vi "Begin.vi"(8 "error in":errorcluster) -> (0 "error out":errorcluster)   [LabVIEW 2015]
doc: "Called before other user functions, this VI is expected to open initial I/O refnums, load in file data, and do all program initialization. Notice that the <B>error out</B> terminal is simply used for data flow. Wiring it to other structures or subVIs ensures that this VI runs first."
uses:
  <vilib>/Rock Robotics/SystemInterfaces/DIO/FPGA_DIOPWMChannel.ctl
  <vilib>/Rock Robotics/WPI/DriverStation/WPI_DriverStationRobotMode2.ctl
  <vilib>/Rock Robotics/WPI/Joystick/WPI_JoystickDeviceEnum.ctl
  <vilib>/Rock Robotics/SystemInterfaces/AI/FPGA_AIChannel.ctl
  <vilib>/Rock Robotics/WPI/SafetyOutput/WPI_SafetyOutputConfigMenu.ctl
  <vilib>/Rock Robotics/SystemInterfaces/DIO/FPGA_DIOChannel.ctl
  <vilib>/Rock Robotics/WPI/Solenoid/WPI_SolenoidChannel.ctl
  <vilib>/Rock Robotics/SystemInterfaces/spilib/spi_bus.ctl
  <vilib>/Rock Robotics/WPI/RobotDrive/WPI_RobotDriveOpen2MotorWithSPARK.vi
  Robot Global Data.vi
  <vilib>/Rock Robotics/Network Tables/NT Write String Array.vi
  <vilib>/Rock Robotics/WPI/MotorControl/WPI_MotorControlOpen SPARK.vi
  <vilib>/Rock Robotics/WPI/Counter/WPI_CounterDigitalInputToDigitalSource.vi
  <vilib>/Rock Robotics/WPI/Solenoid/WPI_SolenoidOpenDouble.vi
  NavX/navX Library v2.lvlib
  ArmController/ArmController.lvlib
  <vilib>/Rock Robotics/WPI/Solenoid/WPI_SolenoidSetEnum.vi
  <vilib>/Rock Robotics/WPI/Solenoid/WPI_SolenoidValue.ctl
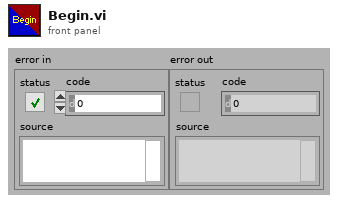
[diagram p1: front panel]
types:
  T1 = typedef "WPI_SafetyOutputConfigMenu.ctl" = enum16{"Enable", "Disable"}
  T2 = typedef "WPI_SolenoidChannel.ctl" = enum8{"Solenoid 0", "Solenoid 1", "Solenoid 2", "Solenoid 3", "Solenoid 4", "Solenoid 5", "Solenoid 6", "Solenoid 7", "Invalid"}
  T3 = typedef "FPGA_DIOChannel.ctl" = enum8{"DIO 0", "DIO 1", "DIO 2", "DIO 3", "DIO 4", "DIO 5", "DIO 6", "DIO 7", "DIO 8", "DIO 9", "DIO MXP 0", "DIO MXP 1", "DIO MXP 2", "DIO MXP 3", "DIO MXP 4", "DIO MXP 5", "DIO MXP 6", "DIO MXP 7", "DIO MXP 8", "DIO MXP 9", "DIO MXP 10", "DIO MXP 11", "DIO MXP 12", "DIO MXP 13", "DIO MXP 14", "DIO MXP 15", "Invalid"}
  T4 = typedef "FPGA_AIChannel.ctl" = enum8{"AI 0", "AI 1", "AI 2", "AI 3", "AI MXP 0", "AI MXP 1", "AI MXP 2", "AI MXP 3", "Invalid"}
  T5 = cluster{"proportional gain (Kc)":dbl, "integral time (Ti, min)":dbl, "derivative time (Td, min)":dbl}
  T6 = typedef "FPGA_DIOPWMChannel.ctl" = enum8{"PWM 0", "PWM 1", "PWM 2", "PWM 3", "PWM 4", "PWM 5", "PWM 6", "PWM 7", "PWM 8", "PWM 9", "PWM MXP 0", "PWM MXP 1", "PWM MXP 2", "PWM MXP 3", "PWM MXP 4", "PWM MXP 5", "PWM MXP 6", "PWM MXP 7", "PWM MXP 8", "PWM MXP 9", "Invalid"}
  T7 = typedef "WPI_JoystickDeviceEnum.ctl" = enum16{"USB 0", "USB 1", "USB 2", "USB 3", "USB 4", "USB 5"}
  T8 = typedef "WPI_DriverStationRobotMode2.ctl" = enum16{"Autonomous Disabled", "Autonomous Enabled", "Teleop Disabled", "Teleop Enabled", "Disconnected", "Finish", "Test Disabled", "Test Enabled", "Emergency Stopped"}
  T9 = typedef "WPI_SolenoidValue.ctl" = enum16{"Off", "On", "Forward", "Reverse"}
  T10 = typedef "WPI_RobotDriveDevRef.ctl" = cluster{"DevStatus":errorcluster, "Motors[]":T11[], "Square Inputs":bool, "Max Output":dbl}
  T11 = typedef "WPI_MotorControlDeviceRef.ctl" = cluster{"DeviceStatus":errorcluster, "Type":T12, "PWM":cluster{"PWM Channel":T6, "DeadBand":T13}, "CAN":cluster{"Device Number":u8, "Control Mode":T14, "Semaphore":T15, "Max Vout":dbl, "TalonSRX Control Mode":T16}, "Invert":bool}
  T12 = typedef "WPI_MotorControlType.ctl" = enum16{"PWM", "CAN", "CANTalonSRX"}
  T13 = typedef "WPI_PWMDeadband.ctl" = cluster{"Name":string, "maxPositivePwm":i32, "minPositivePwm":i32, "centerPwm":i32, "maxNegativePwm":i32, "minNegativePwm":i32, "angularRange":u16}
  T14 = typedef "WPI_CANJaguar_ControlMode.ctl" = enum8{"Percent VBus", "Current", "Speed", "Position", "Voltage"}
  T15 = typedef "Semaphore RefNum" = refnum<k1>
  T16 = typedef "WPI_CANTalonSRX_APIControlMode.ctl" = enum8{"Percent VBus", "Speed", "Position", "Slave", "Unchanged / Invalid", "Voltage Compensation", "Current", "Motion Profile"}
  T17 = typedef "WPI_SolenoidDevRef.ctl" = cluster{"DevStatus":errorcluster, "Pneumatics Control Module":u8, "Forward Solenoid Channel":T2, "Reverse Solenoid Channel":T2}
  T18 = typedef "WPI_ServoDeviceRef.ctl" = cluster{"DeviceStatus":errorcluster, "PWM Channel":T6, "DeadBand":T13}
  T19 = typedef "WPI_JoystickDevRef.ctl" = cluster{"Device":T7}
  T20 = typedef "spi_bus.ctl" = enum16{"SPI On-Board, CS0", "SPI On-Board, CS1", "SPI On-Board, CS2", "SPI On-Board, CS3", "SPI MXP", "Invalid"}
  T21 = typedef "navX Library v2.lvlib/Z900_navX_DeviceTypeDef.ctl" = cluster{"Interface":cluster{"Protocol":T22, "Update Rate (4Hz-60Hz)":u8, "navX Open TypeDef":variant}, "Notify Packet":refnum<notifier>, "Loop VI Refnum":refnum<vi>, "Ready to Close Occurrence Refnum":refnum<k4>}
  T22 = typedef "navX Library v2.lvlib/Z900_navX_ProtocolTypeDef.ctl" = enum16{"SERIAL", "I2C", "SPI"}
  T23 = typedef "WPI_DigitalInputDevRef.ctl" = cluster{"DevStatus":errorcluster, "DIO Channel":T3}
  T24 = typedef "FPGA_CounterEncoderSourceConvertionLVSourceType.ctl" = cluster{"DevStatus":errorcluster, "AnalogTriggerMode?":bool, "DigitalMode":cluster{"DIO Channel":T25}, "AnalogTriggerMode":cluster{"AnalogTriggerIndex":T26, "OutputType":T27}}
  T25 = typedef "FPGA_DIODigitalSourceChannel.ctl" = enum8{"DIO 0", "DIO 1", "DIO 2", "DIO 3", "DIO 4", "DIO 5", "DIO 6", "DIO 7", "DIO 8", "DIO 9", "DIO MXP 0", "DIO MXP 1", "DIO MXP 2", "DIO MXP 3", "DIO MXP 4", "DIO MXP 5", "DIO MXP 6", "DIO MXP 7", "DIO MXP 8", "DIO MXP 9", "DIO MXP 10", "DIO MXP 11", "DIO MXP 12", "DIO MXP 13", "DIO MXP 14", "DIO MXP 15", "Disabled"}
  T26 = typedef "FPGA_AnalogTriggerIndex.ctl" = enum8{"Trig 0", "Trig 1", "Trig 2", "Trig 3", "Trig 4", "Trig 5", "Trig 6", "Trig 7", "Invalid"}
  T27 = typedef "FPGA_AnalogTriggerOutType.ctl" = enum16{"InWindow", "TriggerState", "Rising", "Falling"}
  T28 = typedef "WPI_EncoderDevRef.ctl" = cluster{"DevStatus":errorcluster, "EncoderIndex":T29, "CounterIndex":T30, "DistancePerCount":dbl, "Decoding Type":T31}
  T29 = typedef "FPGA_EncoderIdx.ctl" = enum8{"Enc 0", "Enc 1", "Enc 2", "Enc 3", "Enc 4", "Enc 5", "Enc 6", "Enc 7", "Invalid"}
  T30 = typedef "FPGA_CounterCtrSystemIndex.ctl" = enum8{"Ctr 0", "Ctr 1", "Ctr 2", "Ctr 3", "Ctr 4", "Ctr 5", "Ctr 6", "Ctr 7", "Invalid"}
  T31 = typedef "WPI_EncoderType.ctl" = enum16{"1x", "2x", "4x"}
  T32 = typedef "WPI_PotentiometerDevRef.ctl" = cluster{"DevStatus":errorcluster, "Analog Channel":T4, "Invert Output":bool}
  T33 = typedef "ArmController.lvlib/ArmRef.ctl" = cluster{"Pot":T32, "ArmMotor":T11, "Queue":refnum<queue>, "Setpoint":dbl, "Manual":bool, "output range":cluster{"output high":dbl, "output low":dbl}, "PID gains":cluster{"proportional gain (Kc)":dbl, "integral time (Ti, min)":dbl, "derivative time (Td, min)":dbl}}
  T34 = typedef "WPI_AnalogChannelDevRef.ctl" = cluster{"DevStatus":errorcluster, "Analog Channel":T4}
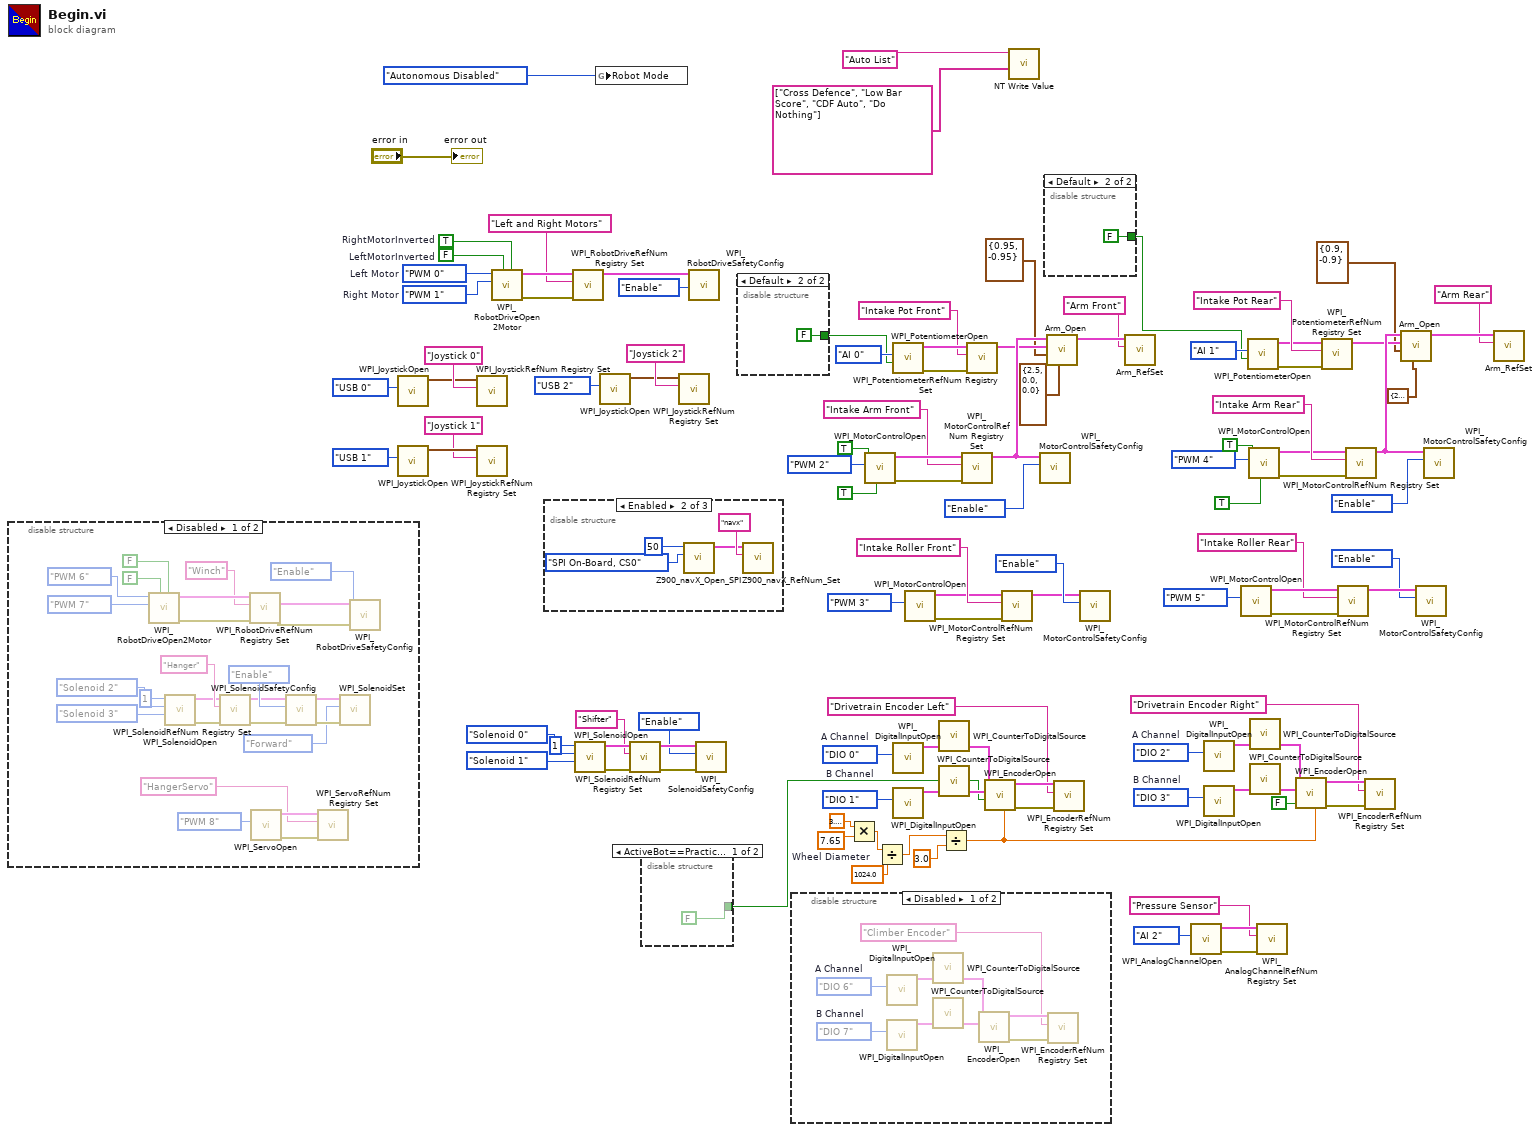
[diagram p0: block diagram]
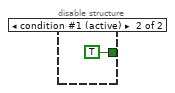
[diagram p3: hidden frame]
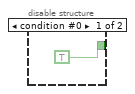
[diagram p4: hidden frame]
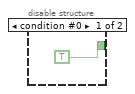
[diagram p5: hidden frame]
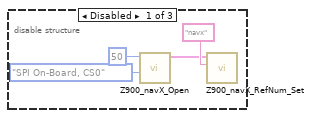
[diagram p6: hidden frame]
diagram:
  w19 = 7.65  # Wheel Diameter
  w30 = FPGA_DIOChannel."DIO 3"  # B Channel
  w29 = FPGA_DIOChannel."DIO 2"  # A Channel
  w38 = FPGA_DIOChannel."DIO 1"  # B Channel
  w37 = FPGA_DIOChannel."DIO 0"  # A Channel
  w104 = FPGA_DIOPWMChannel."PWM 1"  # Right Motor
  w105 = FPGA_DIOPWMChannel."PWM 0"  # Left Motor
  w109 = FALSE  # LeftMotorInverted
  w110 = TRUE  # RightMotorInverted
  n1 = disable-structure shown="Disabled" {
    frame Disabled {
      n2 = call-poly <vilib>:"WPI_RobotDriveOpen2Motor.vi"("Right Motor Inverted"=FALSE, "Left Motor Inverted"=FALSE, "Right Motor"=FPGA_DIOPWMChannel."PWM 7", "Left Motor"=FPGA_DIOPWMChannel."PWM 6") -> ("error out"=w122:errorcluster, "RobotDriveDevRef"=w123:T10)  [unwired: 6 in]
      n3 = call-poly <vilib>:"WPI_SolenoidOpen.vi"("Reverse Solenoid Channel"=WPI_SolenoidChannel."Solenoid 3", "Forward Solenoid Channel"=WPI_SolenoidChannel."Solenoid 2", "Pneumatics Control Module (0)"=u8 1) -> ("error out"=w129:errorcluster, "SolenoidDevRef"=w128:T17)  [unwired: 7 in]
      n4 = call <vilib>:"WPI_SolenoidRefNum Registry Set.vi"("error in (no error)"=w129, "refnum name"="Hanger", "SolenoidDevRef"=w128) -> ("error out"=w132:errorcluster, "SolenoidDevRef"=w131:T17)  [unwired: 7 in]
      n5 = call <vilib>:"WPI_RobotDriveRefNum Registry Set.vi"("error in (no error)"=w122, "refnum name"="Winch", "RobotDriveDevRef"=w123) -> ("error out"=w118:errorcluster, "RobotDriveDevRef"=w119:T10)  [unwired: 7 in]
      n6 = call <vilib>:"WPI_ServoOpen.vi"("PWM Channel"=FPGA_DIOPWMChannel."PWM 8") -> ("error out"=w114:errorcluster, "ServoDeviceRef"=w113:T18)  [unwired: 9 in]
      n7 = call <vilib>:"WPI_SolenoidSafetyConfig.vi"("error in (no error)"=w132, "mode"=WPI_SafetyOutputConfigMenu."Enable", "SolenoidDevRef"=w131) -> ("error out"=w117:errorcluster, "SolenoidDevRef"=w116:T17)  [unwired: 7 in]
      n8 = call <vilib>:"WPI_ServoRefNum Registry Set.vi"("error in (no error)"=w114, "refnum name"="HangerServo", "ServoDeviceRef"=w113) -> ()  [unwired: 7 in, 2 out]
      n9 = call-poly <vilib>:"WPI_SolenoidSet.vi"("error in (no error)"=w117, "Value"=WPI_SolenoidValue."Forward", "SolenoidDevRef"=w116) -> ()  [unwired: 7 in, 2 out]
      n10 = call <vilib>:"WPI_RobotDriveSafetyConfig.vi"("error in (no error)"=w118, "mode"=WPI_SafetyOutputConfigMenu."Enable", "RobotDriveDevRef"=w119) -> ()  [unwired: 7 in, 2 out]
    }
    frame Enabled {
    }
  }
  n11 = call <vilib>:"WPI_JoystickOpen.vi"("JoystickDevice"=WPI_JoystickDeviceEnum."USB 0") -> ("JoystickDevRef"=w99:T19)  [unwired: 10 in]
  n12 = call <vilib>:"WPI_JoystickOpen.vi"("JoystickDevice"=WPI_JoystickDeviceEnum."USB 1") -> ("JoystickDevRef"=w93:T19)  [unwired: 10 in]
  n13 = call <vilib>:"WPI_JoystickRefNum Registry Set.vi"("refnum name"="Joystick 0", "JoystickDevRef"=w99) -> ()  [unwired: 8 in, 2 out]
  n14 = call <vilib>:"WPI_JoystickRefNum Registry Set.vi"("refnum name"="Joystick 1", "JoystickDevRef"=w93) -> ()  [unwired: 8 in, 2 out]
  n15 = call-poly <vilib>:"WPI_RobotDriveOpen2Motor.vi"("Right Motor Inverted"=w110, "Left Motor Inverted"=w109, "Right Motor"=w104, "Left Motor"=w105) -> ("error out"=w106:errorcluster, "RobotDriveDevRef"=w108:T10)  [unwired: 1 in, 5 out]
  n16 = disable-structure shown="Enabled" {
    frame Disabled {
      n17 = call-poly "Z900_navX_Open.vi"("SPI Bus"=spi_bus."SPI On-Board, CS0", "Update Rate (4Hz-60Hz)"=u8 50) -> ("navX Device"=w139:T21)  [unwired: 8 in, 1 out]
      n18 = call "Z900_navX_RefNum_Set.vi"("refnum name"="navx", "navX Device"=w139) -> ()  [unwired: 8 in, 2 out]
    }
    frame Enabled {
      n19 = call "Z900_navX_Open_SPI.vi"("SPI Bus"=spi_bus."SPI On-Board, CS0", "Update Rate (4Hz-60Hz)"=u8 50) -> ("navX Device"=w141:T21)  [unwired: 8 in, 1 out]
      n20 = call "Z900_navX_RefNum_Set.vi"("refnum name"="navx", "navX Device"=w141) -> ()  [unwired: 8 in, 2 out]
    }
    frame Disabled {
    }
  }
  n21 = call <vilib>:"WPI_RobotDriveRefNum Registry Set.vi"("error in (no error)"=w106, "refnum name"="Left and Right Motors", "RobotDriveDevRef"=w108) -> ("RobotDriveDevRef"=w103:T10)  [unwired: 1 in, 7 out]
  n22 = call-poly <vilib>:"WPI_SolenoidOpen.vi"("Reverse Solenoid Channel"=WPI_SolenoidChannel."Solenoid 1", "Forward Solenoid Channel"=WPI_SolenoidChannel."Solenoid 0", "Pneumatics Control Module (0)"=u8 1) -> ("error out"=w11:errorcluster, "SolenoidDevRef"=w12:T17)  [unwired: 7 in]
  n23 = global write "Robot Global Data.vi" "Robot Mode"(WPI_DriverStationRobotMode2."Autonomous Disabled" ("Robot Mode")) -> ()
  n24 = call <vilib>:"WPI_JoystickOpen.vi"("JoystickDevice"=WPI_JoystickDeviceEnum."USB 2") -> ("JoystickDevRef"=w90:T19)  [unwired: 10 in]
  n25 = call <vilib>:"WPI_SolenoidRefNum Registry Set.vi"("error in (no error)"=w11, "refnum name"="Shifter", "SolenoidDevRef"=w12) -> ("error out"=w8:errorcluster, "SolenoidDevRef"=w9:T17)  [unwired: 7 in]
  n26 = disable-structure shown="ActiveBot==Practice" {
    disable-tunnel: [FALSE ("Invert Output") TRUE ("Invert Output")] -> w1
    frame condition #0 {
    }
    frame condition #1 (active) {
    }
  }
  n27 = call <vilib>:"WPI_JoystickRefNum Registry Set.vi"("refnum name"="Joystick 2", "JoystickDevRef"=w90) -> ()  [unwired: 8 in, 2 out]
  n28 = call <vilib>:"WPI_RobotDriveSafetyConfig.vi"("mode"=WPI_SafetyOutputConfigMenu."Enable", "RobotDriveDevRef"=w103) -> ()  [unwired: 8 in, 2 out]
  n29 = call <vilib>:"WPI_SolenoidSafetyConfig.vi"("error in (no error)"=w8, "mode"=WPI_SafetyOutputConfigMenu."Enable", "SolenoidDevRef"=w9) -> ()  [unwired: 7 in, 2 out]
  n30 = disable-structure shown="Default" {
    disable-tunnel: [TRUE ("Invert Output") FALSE ("Invert Output")] -> w3
    frame condition #0 {
    }
    frame condition #1 (active) {
    }
  }
  n31 = disable-structure shown="Disabled" {
    frame Disabled {
      w157 = FPGA_DIOChannel."DIO 7"  # B Channel
      w156 = FPGA_DIOChannel."DIO 6"  # A Channel
      n32 = call <vilib>:"WPI_DigitalInputOpen.vi"("DIO Channel"=w156) -> ("DigitalInputDevRef"=w154:T23)  [unwired: 1 in, 9 out]
      n33 = call <vilib>:"WPI_DigitalInputOpen.vi"("DIO Channel"=w157) -> ("DigitalInputDevRef"=w155:T23)  [unwired: 1 in, 9 out]
      n34 = call-poly <vilib>:"WPI_CounterToDigitalSource.vi"("DigitalInputDevRef"=w154) -> ("Digital Source"=w153:T24)  [unwired: 6 out]
      n35 = call-poly <vilib>:"WPI_CounterToDigitalSource.vi"("DigitalInputDevRef"=w155) -> ("Digital Source"=w149:T24)  [unwired: 6 out]
      n36 = call <vilib>:"WPI_EncoderOpen.vi"("BSource"=w149, "ASource"=w153) -> ("error out"=w151:errorcluster, "EncoderDevRef"=w152:T28)  [unwired: 6 in, 2 out]
      n37 = call <vilib>:"WPI_EncoderRefNum Registry Set.vi"("error in (no error)"=w151, "refnum name"="Climber Encoder", "EncoderDevRef"=w152) -> ()  [unwired: 7 in, 2 out]
    }
    frame Enabled {
    }
  }
  n38 = Multiply(x=3.141592653589793, y=w19) -> (x*y=w18:dbl)
  n39 = call-poly <vilib>:"WPI_MotorControlOpen.vi"("Invert"=TRUE, "Eliminate Deadband"=TRUE, "PWM Channel"=FPGA_DIOPWMChannel."PWM 2") -> ("error out"=w79:errorcluster, "MotorControlDeviceRef"=w78:T11)  [unwired: 7 in]
  n40 = Divide(x=w18, y=1024.0) -> (x/y=w17:dbl)
  n41 = call <vilib>:"WPI_PotentiometerOpen.vi"("Invert Output"=w3, "Analog Channel"=FPGA_AIChannel."AI 0") -> ("error out"=w86:errorcluster, "PotDevRef"=w87:T32)  [unwired: 8 in]
  n42 = call <vilib>:"WPI_DigitalInputOpen.vi"("DIO Channel"=w37) -> ("DigitalInputDevRef"=w35:T23)  [unwired: 1 in, 9 out]
  n43 = call <vilib>:"WPI_DigitalInputOpen.vi"("DIO Channel"=w38) -> ("DigitalInputDevRef"=w36:T23)  [unwired: 1 in, 9 out]
  n44 = call-poly <vilib>:"WPI_MotorControlOpen.vi"("PWM Channel"=FPGA_DIOPWMChannel."PWM 3") -> ("error out"=w71:errorcluster, "MotorControlDeviceRef"=w72:T11)  [unwired: 9 in]
  n45 = call-poly <vilib>:"WPI_CounterToDigitalSource.vi"("DigitalInputDevRef"=w35) -> ("Digital Source"=w34:T24)  [unwired: 6 out]
  n46 = call-poly <vilib>:"WPI_CounterToDigitalSource.vi"("DigitalInputDevRef"=w36) -> ("Digital Source"=w21:T24)  [unwired: 6 out]
  n47 = Divide(x=w17, y=3.0 ("x")) -> (x/y=w15:dbl)
  n48 = call <vilib>:"WPI_MotorControlRefNum Registry Set.vi"("error in (no error)"=w79, "refnum name"="Intake Arm Front", "MotorControlDevRef"=w78) -> ("MotorControlDevRef"=w58:T11)  [unwired: 7 in, 1 out]
  n49 = call <vilib>:"WPI_PotentiometerRefNum Registry Set.vi"("error in (no error)"=w86, "refnum name"="Intake Pot Front", "PotDevRef"=w87) -> ("PotDevRef"=w57:T32)  [unwired: 7 in, 1 out]
  n50 = call <vilib>:"WPI_EncoderOpen.vi"("DistancePerCount"=w15, "Invert Direction (False)"=w1, "BSource"=w21, "ASource"=w34) -> ("error out"=w32:errorcluster, "EncoderDevRef"=w33:T28)  [unwired: 4 in, 2 out]
  n51 = call <vilib>:"WPI_MotorControlRefNum Registry Set.vi"("error in (no error)"=w71, "refnum name"="Intake Roller Front", "MotorControlDevRef"=w72) -> ("MotorControlDevRef"=w74:T11)  [unwired: 7 in, 1 out]
  n52 = call-poly <vilib>:"NT Write Value.vi"("String Array"=string[] ["Cross Defence", "Low Bar Score", "CDF Auto", "Do Nothing"], "Name"="Auto List") -> ()  [unwired: 9 in, 1 out]
  n53 = call <vilib>:"WPI_MotorControlSafetyConfig.vi"("mode"=WPI_SafetyOutputConfigMenu."Enable", "MotorControlDevRef"=w58) -> ()  [unwired: 8 in, 2 out]
  n54 = disable-structure shown="Default" {
    disable-tunnel: [TRUE ("Invert Output") FALSE ("Invert Output")] -> w2
    frame condition #0 {
    }
    frame condition #1 (active) {
    }
  }
  n55 = call "Arm_Open.vi"("PID gains"=T5 {"proportional gain (Kc)"=2.5, "integral time (Ti, min)"=0.0, "derivative time (Td, min)"=0.0}, "output range"=cluster{"output high":dbl, "output low":dbl} {"output high"=0.95, "output low"=-0.95}, "PotDevRef"=w57, "ArmMotor"=w58) -> ("ArmRef"=w54:T33)  [unwired: 7 in]
  n56 = call <vilib>:"WPI_EncoderRefNum Registry Set.vi"("error in (no error)"=w32, "refnum name"="Drivetrain Encoder Left", "EncoderDevRef"=w33) -> ()  [unwired: 7 in, 2 out]
  n57 = call <vilib>:"WPI_MotorControlSafetyConfig.vi"("mode"=WPI_SafetyOutputConfigMenu."Enable", "MotorControlDevRef"=w74) -> ()  [unwired: 8 in, 2 out]
  n58 = call "Arm_RefSet.vi"("refnum name"="Arm Front", "ArmRef in"=w54) -> ()  [unwired: 8 in, 2 out]
  n59 = call <vilib>:"WPI_AnalogChannelOpen.vi"("Analog Channel"=FPGA_AIChannel."AI 2") -> ("error out"=w40:errorcluster, "AIDeviceRef"=w41:T34)  [unwired: 9 in]
  n60 = call <vilib>:"WPI_DigitalInputOpen.vi"("DIO Channel"=w29) -> ("DigitalInputDevRef"=w26:T23)  [unwired: 1 in, 9 out]
  n61 = call <vilib>:"WPI_DigitalInputOpen.vi"("DIO Channel"=w30) -> ("DigitalInputDevRef"=w27:T23)  [unwired: 1 in, 9 out]
  n62 = call-poly <vilib>:"WPI_MotorControlOpen.vi"("PWM Channel"=FPGA_DIOPWMChannel."PWM 5") -> ("error out"=w68:errorcluster, "MotorControlDeviceRef"=w67:T11)  [unwired: 9 in]
  n63 = call <vilib>:"WPI_PotentiometerOpen.vi"("Invert Output"=w2, "Analog Channel"=FPGA_AIChannel."AI 1") -> ("error out"=w83:errorcluster, "PotDevRef"=w82:T32)  [unwired: 8 in]
  n64 = call-poly <vilib>:"WPI_MotorControlOpen.vi"("Invert"=TRUE, "Eliminate Deadband"=TRUE, "PWM Channel"=FPGA_DIOPWMChannel."PWM 4") -> ("error out"=w60:errorcluster, "MotorControlDeviceRef"=w61:T11)  [unwired: 7 in]
  n65 = call-poly <vilib>:"WPI_CounterToDigitalSource.vi"("DigitalInputDevRef"=w26) -> ("Digital Source"=w25:T24)  [unwired: 6 out]
  n66 = call-poly <vilib>:"WPI_CounterToDigitalSource.vi"("DigitalInputDevRef"=w27) -> ("Digital Source"=w28:T24)  [unwired: 6 out]
  n67 = call <vilib>:"WPI_AnalogChannelRefNum Registry Set.vi"("error in (no error)"=w40, "refnum name"="Pressure Sensor", "AIDeviceRef"=w41) -> ()  [unwired: 7 in, 2 out]
  n68 = call <vilib>:"WPI_EncoderOpen.vi"("DistancePerCount"=w15, "Invert Direction (False)"=FALSE, "BSource"=w28, "ASource"=w25) -> ("error out"=w23:errorcluster, "EncoderDevRef"=w24:T28)  [unwired: 4 in, 2 out]
  n69 = call <vilib>:"WPI_PotentiometerRefNum Registry Set.vi"("error in (no error)"=w83, "refnum name"="Intake Pot Rear", "PotDevRef"=w82) -> ("PotDevRef"=w55:T32)  [unwired: 7 in, 1 out]
  n70 = call <vilib>:"WPI_MotorControlRefNum Registry Set.vi"("error in (no error)"=w68, "refnum name"="Intake Roller Rear", "MotorControlDevRef"=w67) -> ("MotorControlDevRef"=w65:T11)  [unwired: 7 in, 1 out]
  n71 = call <vilib>:"WPI_MotorControlRefNum Registry Set.vi"("error in (no error)"=w60, "refnum name"="Intake Arm Rear", "MotorControlDevRef"=w61) -> ("MotorControlDevRef"=w56:T11)  [unwired: 7 in, 1 out]
  n72 = call <vilib>:"WPI_EncoderRefNum Registry Set.vi"("error in (no error)"=w23, "refnum name"="Drivetrain Encoder Right", "EncoderDevRef"=w24) -> ()  [unwired: 7 in, 2 out]
  n73 = call "Arm_Open.vi"("PID gains"=T5 {"proportional gain (Kc)"=2.5, "integral time (Ti, min)"=0.0, "derivative time (Td, min)"=0.0}, "output range"=cluster{"output high":dbl, "output low":dbl} {"output high"=0.9, "output low"=-0.9}, "PotDevRef"=w55, "ArmMotor"=w56) -> ("ArmRef"=w53:T33)  [unwired: 7 in]
  n74 = call <vilib>:"WPI_MotorControlSafetyConfig.vi"("mode"=WPI_SafetyOutputConfigMenu."Enable", "MotorControlDevRef"=w65) -> ()  [unwired: 8 in, 2 out]
  n75 = call <vilib>:"WPI_MotorControlSafetyConfig.vi"("mode"=WPI_SafetyOutputConfigMenu."Enable", "MotorControlDevRef"=w56) -> ()  [unwired: 8 in, 2 out]
  n76 = call "Arm_RefSet.vi"("refnum name"="Arm Rear", "ArmRef in"=w53) -> ()  [unwired: 8 in, 2 out]
  "error out" <- "error in"
